vi "CreateSpecialVIWrapper.vi"(8 "error in (no error)":errorcluster) -> (0 "error out":errorcluster)   [LabVIEW 2020, in "WebServiceImporter.lvlib" / "VI Generator.lvlib"]
uses:
  <vilib>/Platform/WebService/VI Generator/VI Generator.lvlib
  <vilib>/Platform/WebService/Error Handling/Error/Context Name.ctl
  <vilib>/Platform/WebService/Error Handling/Error/Error Number.ctl
  <vilib>/Platform/WebService/Error Handling/Error Handling.lvlib
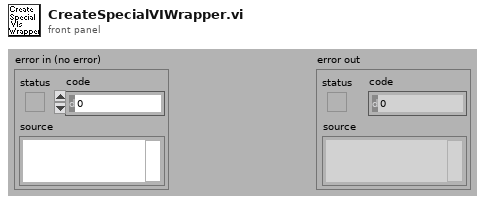
[diagram p1: front panel]
types:
  T1 = typedef "WebServiceImporter.lvlib/Error Handling.lvlib/Error Number.ctl" = u16
  T2 = typedef "WebServiceImporter.lvlib/Error Handling.lvlib/Context Name.ctl" = u16
  T3 = typedef "WebServiceImporter.lvlib/Error Handling.lvlib/Context.ctl" = cluster{"name":T2, "value":string}[]
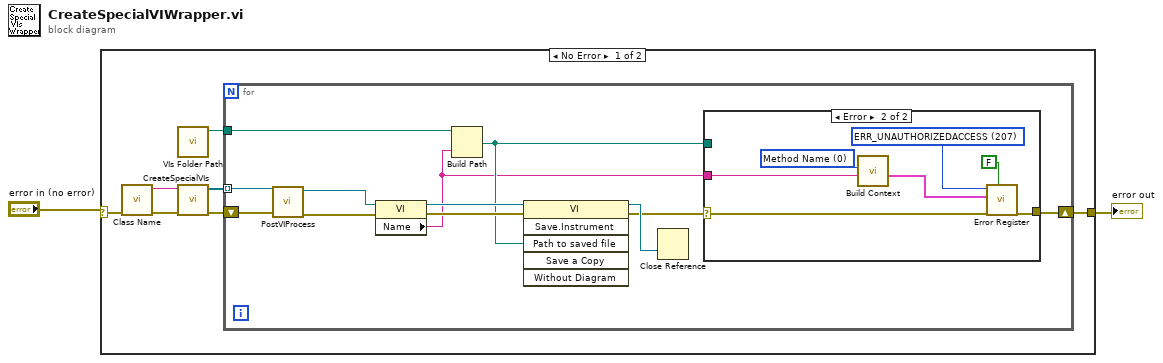
[diagram p0: block diagram]
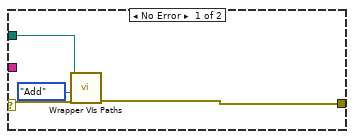
[diagram p2: hidden frame]
diagram:
  n1 = case shown="No Error" "error in (no error)" {
    selector: "error in (no error)" -> [w9 w32]
    tunnel: [w4 w32] -> w1
    frame No Error {
      n2 = call <vilib>:"Class Name.vi"("error in (no error)"=w9) -> ("error out"=w8:errorcluster, "Class Name (out)"=w7:string)  [unwired: 9 in]
      n3 = call <vilib>:"VIs Folder Path.vi"() -> ("Path 2"=w3:path)  [unwired: 10 in, 1 out]
      n4 = call <vilib>:"CreateSpecialVIs.vi"("Class Name"=w7, "error in (no error)"=w8) -> ("Created VIs"=w6:refnum<vi>[], "error out"=w5:errorcluster)  [unwired: 7 in]
      n5 = for {
        tunnel: w6 -> [w13] mode=indexing
        shift-right: [w16] -> w4
        shift-left: w5 -> [w12]
        tunnel: w3 -> [w21]
        n6 = call <vilib>:"PostVIProcess.vi"("error in (no error)"=w12, "VI Refnum"=w13) -> ("error out"=w11:errorcluster, "VI Refnum Out"=w10:refnum<vi>)  [unwired: 8 in]
        n7 = property class="VI"(reference=w10, error in=w11) -> (reference out=w20:refnum<vi>, error out=w19:errorcluster, "Name"=w15:string)
        n8 = Build Path(base path=w21, name or relative path=w15) -> (appended path=w17:path)
        n9 = invoke class="VI" method="Save.Instrument"(reference=w20, error in=w19, "Path to saved file"=w17) -> (reference out=w18:refnum<vi>, error out=w14:errorcluster)  [unwired: 3 in, 4 out]
        n10 = Close Reference(reference=w18) -> ()  [unwired: 1 in, 1 out]
        n11 = case shown="Error" w14 {
          selector: w14 -> [w25 w31]
          tunnel: w17 -> [w23 _]
          tunnel: [w22 w31] -> w16
          tunnel: w15 -> [_ w26]
          frame No Error {
            n12 = call <vilib>:"Wrapper VIs Paths.vi"("error in (no error)"=w25, "Op"=enum16{"Get", "Add", "Clear"}."Add", "Path"=w23) -> ("error out"=w22:errorcluster)  [unwired: 7 in, 1 out]
          }
          frame Error {
            w27 = T1 207 items=["ERR_NOERROR"=0, "ERR_ACCESS_OUTPUTFOLDER"=1, "ERR_INVALID_LIBRARYNAME"=2, "ERR_CREATE_VIWRAPPER"=3, "ERR_UNKNOWN"=201, "ERR_BAD_ARGUMENT"=202, "ERR_URL_NOTFOUND_BADWSDL"=203, "ERR_BADLYFORMATTEDURL"=204, "ERR_BADHOSTNAME"=205, "ERR_BADDIRECTORY"=206, "ERR_UNAUTHORIZEDACCESS"=207] ("Error Number")
            w30 = T2 0 items=["Method Name", "Parameter Name", "VI Name", "Control Name", "Proxy Dll Path"] ("Context Name")
            n13 = call <vilib>:"Build Context.vi"("Context Value"=w26, "Context Name"=w30) -> ("Context"=w28:T3)  [unwired: 9 in]
            n14 = call <vilib>:"Error Register.vi"("Throw Up?"=FALSE, "Context"=w28, "Error Number"=w27) -> ()  [unwired: 8 in, 1 out]
          }
        }
      }
    }
    frame Error {
    }
  }
  "error out" <- w1
